vi "Desktop Main.vi"() -> ()   [LabVIEW 2014]
uses:
  SubVIs/myRIO/Controls/Switch Schedule.ctl
  SubVIs/myRIO/Controls/Switch Program.ctl
  SubVIs/myRIO/Controls/Action Enum.ctl
  SubVIs/myRIO/Controls/Switch Day.ctl
  SubVIs/Host/Controls/UDP Reference Action Enum.ctl
  SubVIs/myRIO/Controls/myRIO Data.ctl
panel:
  in  "Sync":bool
  in  "Listen":bool=TRUE
  in  "Modify":bool caption="Off"
  in  "Send":bool caption="Off"
  in  "Off":bool
  in  "On":bool
  in  "myRIO IP Address":string="172.22.11.2"
  in  "Delete Buttons":T1
  out "myRIO Time":timestamp format="%<%X\n%x>T"
  out "Index Values":u32[](array[numeric])
  in  "Switch Schedule":T2
  in  "stop":bool
  # "Computer Instructions\n1. See READ ME to properly \n    configure time on NI myRIO.\n2.  Open RT Main.vi and enter\n     your computer IP address.\n3.  Run RT Main.vi\n4.  Specify myRIO IP Address\n      in Desktop Main.vi\n5.   Run Desktop Main.vi\n6.   Click Sync to sync time\n7.   Push On to turn on switch\n8.   Push Off to turn off switch\n9.   Click Modify Schedule to\n      schedule an action.\n10.   Click the Action drop-down\n      to specify Action.\n11.  Enter Time of Action in\n       24-hour format.\n12. Select Day for Action to\n      take place. Choose \"Eee\"\n      for every day.\n13. Click Send Updates to save\n      the schedule.\n\nSmartphone Instructions\n1.  Set up your myRIO for WiFi.\n2.  Install a UDP app for your\n     smartphone.\n3.  Run RT Main.vi.\n3.  Enter the myRIO's IP address\n    into the app.\n4. Send \"on\" or \"off\"\n5. See documentation for more\n    commands."
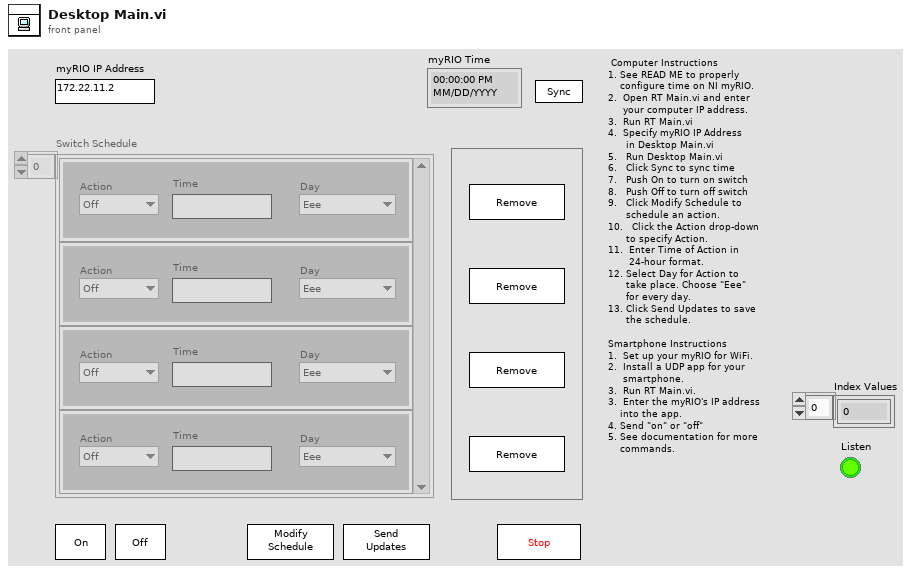
[diagram p1: front panel]
types:
  T1 = cluster{"Remove 0":bool, "Remove 1":bool, "Remove 2":bool, "Remove 3":bool}
  T2 = typedef "Switch Schedule.ctl" = T3[]
  T3 = typedef "Switch Program.ctl" = cluster{"Action":T4, "Time":string, "Day":T5}
  T4 = typedef "Action Enum.ctl" = enum16{"Off", "On"}
  T5 = typedef "Switch Day.ctl" = enum16{"Eee", "Sun", "Mon", "Tue", "Wed", "Thu", "Fri", "Sat"}
  T6 = enum8{"Enabled", "Disabled", "Disabled and Grayed Out"}
  T7 = typedef "UDP Reference Action Enum.ctl" = enum16{"Set", "Get"}
  T8 = typedef "myRIO Data.ctl" = cluster{"Time":timestamp, "Switch Schedule":T2}
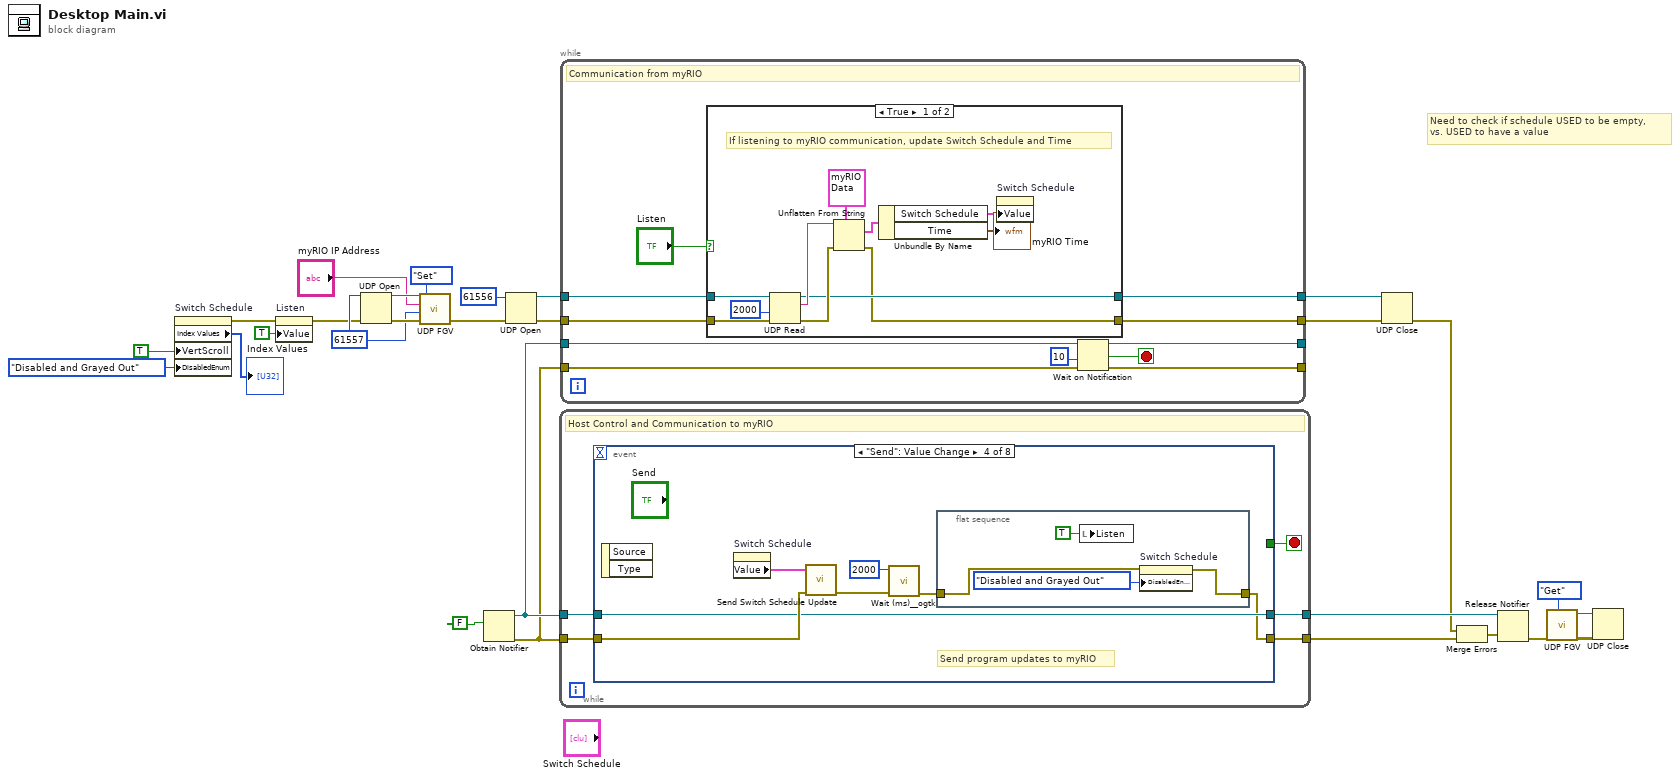
[diagram p0: block diagram]
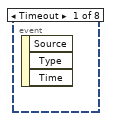
[diagram p2: hidden frame]
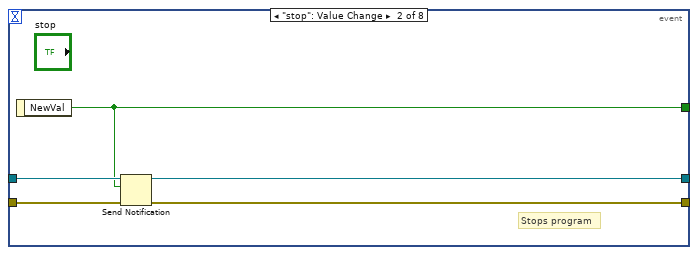
[diagram p3: hidden frame]
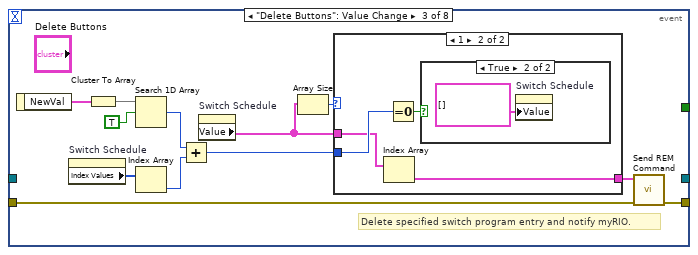
[diagram p4: hidden frame]
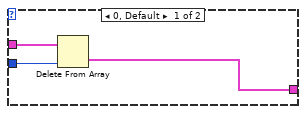
[diagram p5: hidden frame]
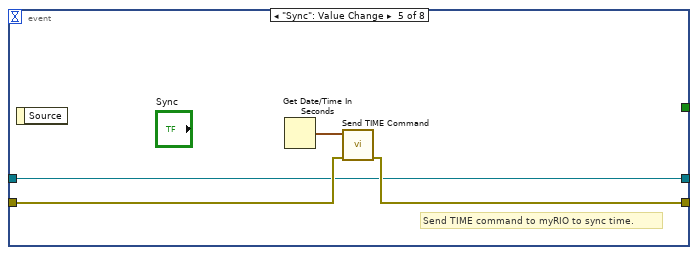
[diagram p7: hidden frame]
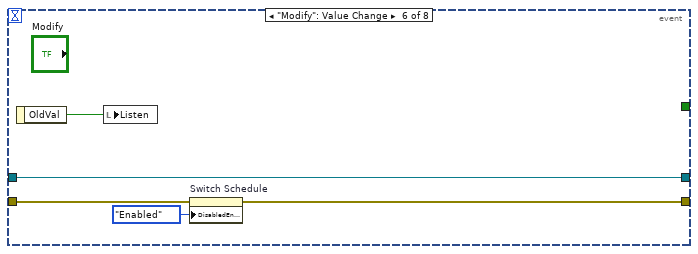
[diagram p8: hidden frame]
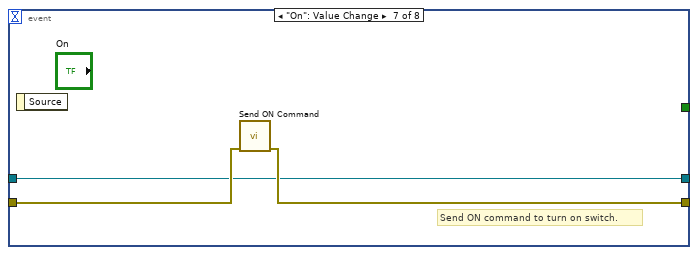
[diagram p9: hidden frame]
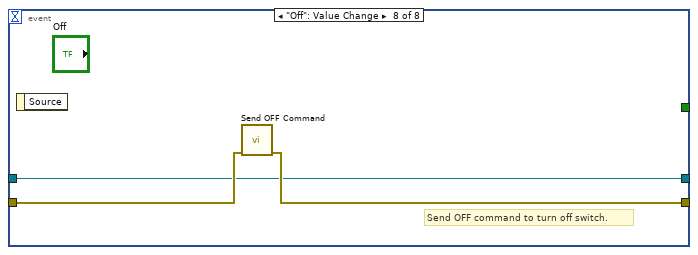
[diagram p10: hidden frame]
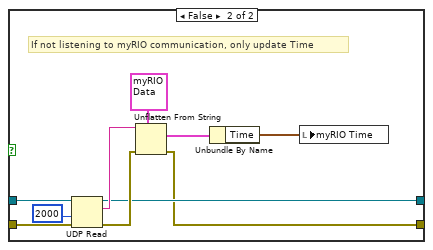
[diagram p11: hidden frame]
diagram:
  w10 = u16 61557 ("port")
  # "Need to check if schedule USED to be empty, \nvs. USED to have a value"
  n1 = property on="Switch Schedule" class="Arr (strict)"("VertScroll"=TRUE ("Vertical Scrollbar Visible"), "DisabledEnum"=T6."Disabled and Grayed Out" ("Disabled")) -> (error out=w3:errorcluster, "Index Values"=→"Index Values":u32[])  [unwired: 2 in, 1 out]
  n2 = property on="Listen" class="Bool (strict)"(error in=w3, "Value"=TRUE ("Listen")) -> (error out=w2:errorcluster)  [unwired: 1 in, 1 out]
  n3 = UDP Open(8:w2, 11:w10) -> (port=w11:refnum<k16>, 0:w12:errorcluster)  [unwired: 3 in, 1 out]
  n4 = call "UDP FGV.vi"("Action"=UDP_Reference_Action_Enum."Set", "error in (no error)"=w12, "Port"=w10, "IP Address"="myRIO IP Address", "connection ID"=w11) -> ("error out"=w13:errorcluster)  [unwired: 3 in, 3 out]
  n5 = Obtain Notifier(notification data type=FALSE) -> (notifier out=w20:refnum<notifier>, error out=w19:errorcluster)  [unwired: 3 in, 1 out]
  n6 = UDP Open(8:w13, 11:u16 61556 ("port")) -> (port=w15:refnum<k16>, 0:w14:errorcluster)  [unwired: 3 in, 1 out]
  n7 = while {
    tunnel: w20 -> [w33]
    tunnel: w19 -> [w32]
    tunnel: [w31] -> w22
    tunnel: [w30] -> w21
    stop <- w29 stop-if-true
    # "Host Control and Communication to myRIO"
    n8 = event shown="[3] \"Send\": Value Change" {
      selector: _ -> [_ _ _ _ _ _ _ _]
      dyn-events: _ -> [_ _ _ _ _ _ _ _]
      timeout: _ -> [_ _ _ _ _ _ _ _]
      tunnel: w33 -> [_ w38 _ w64 w71 w74 w79 w82]
      tunnel: w32 -> [_ w37 w43 w65 w73 w78 w81 w84]
      tunnel: [_ w36 w42 w59 w72 w75 w80 w83] -> w31
      tunnel: [_ w35 _ w64 w71 w74 w79 w82] -> w30
      tunnel: [_ w34 _ _ _ _ _ _] -> w29
      event Timeout {
        n9 = event-data() -> ()  [unwired: 1 in, 3 out]
      }
      event "stop": Value Change {
        # "Stops program"
        n10 = event-data() -> ("NewVal"=w34:bool)  [unwired: 1 in]
        n11 = Send Notification(notification=w34, notifier=w38, error in (no error)=w37) -> (notifier out=w35:refnum<notifier>, error out=w36:errorcluster)
      }
      event "Delete Buttons": Value Change {
        # "Delete specified switch program entry and notify myRIO."
        n12 = event-data() -> ("NewVal"=w50:T1)  [unwired: 1 in]
        n13 = property on="Switch Schedule" class="Arr (strict)"() -> ("Index Values"=w47:u32[])  [unwired: 2 in, 2 out]
        n14 = Cluster To Array(cluster=w50) -> (array=w49:bool[])
        n15 = Search 1D Array(1D array=w49, element=TRUE) -> (index of element=w45:i32)  [unwired: 1 in]
        n16 = Index Array(array=w47) -> (element=w46:u32)  [unwired: 1 in]
        n17 = Add(x=w45, y=w46) -> (x+y=w44:u32)
        n18 = property on="Switch Schedule" class="Arr (strict)"() -> ("Value"=w40:T2)  [unwired: 2 in, 2 out]
        n19 = Array Size(array=w40) -> (size(s)=w39:i32)
        n20 = case shown="1" w39 {
          tunnel: w44 -> [w53 w56]
          tunnel: [w52 w57] -> w41
          tunnel: w40 -> [w51 w55]
          frame 0, Default {
            n21 = Delete From Array(array=w51, index=w53) -> (deleted portion=w52:T3)  [unwired: 1 in, 1 out]
          }
          frame 1 {
            n22 = Index Array(array=w55) -> (element=w57:T3)  [unwired: 1 in]
            n23 = Equal To 0?(x=w56) -> (x = 0?=w54:bool)
            n24 = case shown="True" w54 {
              frame False {
              }
              frame True {
                n25 = property on="Switch Schedule" class="Arr (strict)"("Value"=T2 [] ("t")) -> ()  [unwired: 2 in, 2 out]
              }
            }
          }
        }
        n26 = call "Send REM Command.vi"("error in (no error)"=w43, "Switch Program"=w41) -> ("error out"=w42:errorcluster)  [unwired: 9 in]
      }
      event "Send": Value Change {
        # "Send program updates to myRIO"
        n27 = event-data() -> ()  [unwired: 1 in, 2 out]
        n28 = property on="Switch Schedule" class="Arr (strict)"() -> ("Value"=w63:T2)  [unwired: 2 in, 2 out]
        n29 = call "Send Switch Schedule Update.vi"("error in (no error)"=w65, "Switch Schedule"=w63) -> ("error out"=w62:errorcluster)  [unwired: 9 in]
        n30 = call <userlib>:"Wait (ms)__ogtk.vi"("error in (no error)"=w62, "milliseconds to wait"=u32 2000) -> ("error out"=w60:errorcluster)  [unwired: 8 in, 1 out]
        n31 = flat-sequence {
          tunnel: w60 -> [w67]
          tunnel: [w66] -> w59
          frame #0 {
            n32 = local write "Listen"(TRUE ("Listen")) -> ()
            n33 = property on="Switch Schedule" class="Arr (strict)"(error in=w67, "DisabledEnum"=T6."Disabled and Grayed Out" ("Disabled")) -> (error out=w66:errorcluster)  [unwired: 1 in, 1 out]
          }
        }
      }
      event "Sync": Value Change {
        # "Send TIME command to myRIO to sync time."
        n34 = event-data() -> ()  [unwired: 1 in, 1 out]
        n35 = Get Date/Time In Seconds() -> (seconds since 1Jan1904=w70:timestamp)
        n36 = call "Send TIME Command.vi"("error in (no error)"=w73, "Time Stamp"=w70) -> ("error out"=w72:errorcluster)  [unwired: 9 in]
      }
      event "Modify": Value Change {
        n37 = event-data() -> ("OldVal"=w76:bool)  [unwired: 1 in]
        n38 = local write "Listen"(w76) -> ()
        n39 = property on="Switch Schedule" class="Arr (strict)"(error in=w78, "DisabledEnum"=T6."Enabled" ("Disabled")) -> (error out=w75:errorcluster)  [unwired: 1 in, 1 out]
      }
      event "On": Value Change {
        # "Send ON command to turn on switch."
        n40 = event-data() -> ()  [unwired: 1 in, 1 out]
        n41 = call "Send ON Command.vi"("error in (no error)"=w81) -> ("error out"=w80:errorcluster)  [unwired: 10 in]
      }
      event "Off": Value Change {
        # "Send OFF command to turn off switch."
        n42 = event-data() -> ()  [unwired: 1 in, 1 out]
        n43 = call "Send OFF Command.vi"("error in (no error)"=w84) -> ("error out"=w83:errorcluster)  [unwired: 10 in]
      }
    }
  }
  n44 = while {
    tunnel: w14 -> [w94]
    tunnel: w15 -> [w95]
    tunnel: [w93] -> w27
    tunnel: [w92] -> w26
    tunnel: w20 -> [w91]
    tunnel: w19 -> [w90]
    tunnel: [w89] -> _
    tunnel: [w87] -> _
    stop <- w88 stop-if-true
    # "Communication from myRIO"
    n45 = case shown="True" "Listen" {
      tunnel: w95 -> [w106 w116]
      tunnel: w94 -> [w105 w115]
      tunnel: [w101 w111] -> w93
      tunnel: [w100 w110] -> w92
      frame True {
        # "If listening to myRIO communication, update Switch Schedule and Time"
        n46 = UDP Read(connection ID=w106, timeout ms (25000)=2000, 8:w105) -> (data out=w104:string, error out=w102:errorcluster, 3:w101:refnum<k16>)  [unwired: 1 in, 2 out]
        n47 = Unflatten From String(type=T8 {"Time"=timestamp(0 s since 1904-01-01), "Switch Schedule"=[]} ("myRIO Data"), binary string=w104, error in (no error)=w102) -> (value=w98:T8, error out=w100:errorcluster)  [unwired: 2 in, 1 out]
        n48 = Unbundle By Name(w98) -> ("Switch Schedule"=w96:T2, "Time"=→"myRIO Time":timestamp)
        n49 = property on="Switch Schedule" class="Arr (strict)"("Value"=w96) -> ()  [unwired: 2 in, 2 out]
      }
      frame False {
        # "If not listening to myRIO communication, only update Time"
        n50 = UDP Read(connection ID=w116, timeout ms (25000)=2000, 8:w115) -> (data out=w114:string, error out=w112:errorcluster, 3:w111:refnum<k16>)  [unwired: 1 in, 2 out]
        n51 = Unflatten From String(type=T8 {"Time"=timestamp(0 s since 1904-01-01), "Switch Schedule"=[]} ("myRIO Data"), binary string=w114, error in (no error)=w112) -> (value=w108:T8, error out=w110:errorcluster)  [unwired: 2 in, 1 out]
        n52 = Unbundle By Name(w108) -> ("Time"=w107:timestamp)
        n53 = local write "myRIO Time"(w107) -> ()
      }
    }
    n54 = Wait on Notification(notifier=w91, timeout in ms (-1)=10, error in (no error)=w90) -> (notifier out=w87:refnum<notifier>, notification=w88:bool, error out=w89:errorcluster)  [unwired: 1 in, 1 out]
  }
  n55 = UDP Close(connection ID=w27, 8:w26) -> (error out=w17:errorcluster)  [unwired: 1 out]
  n56 = Merge Errors(w17, w22) -> (w18:errorcluster)
  n57 = Release Notifier(notifier=w21, error in (no error)=w18) -> (error out=w8:errorcluster)  [unwired: 1 in, 2 out]
  n58 = call "UDP FGV.vi"("Action"=UDP_Reference_Action_Enum."Get", "error in (no error)"=w8) -> ("error out"=w6:errorcluster, "connection ID out"=w5:refnum<k16>)  [unwired: 6 in, 2 out]
  n59 = UDP Close(connection ID=w5, 8:w6) -> ()  [unwired: 2 out]
